vi "NI VeriStand - Update Custom Device Flag.vi"(8 "error in (no error)":errorcluster, 10 "Is Custom Device Active?":bool, 11 "Device Ref in":T1 format="%.0x") -> (0 "error out":errorcluster, 3 "Device Ref out":T1 format="%.0x")   [LabVIEW 2020, in "Custom Device API.lvlib"]
doc: "Flags a custom device as active or inactive."
uses:
  <vilib>/NI VeriStand/Custom Device API/Custom Device API.lvlib
  <vilib>/NI VeriStand/Custom Device API/Custom Device Item Ref.ctl
  <vilib>/NI VeriStand/Custom Device API/Custom Device Status.ctl
  380d47f6-5555-4561-b896-d523444e7594.vi
  <vilib>/NI VeriStand/Custom Device API/Custom Device Offline Path.vi
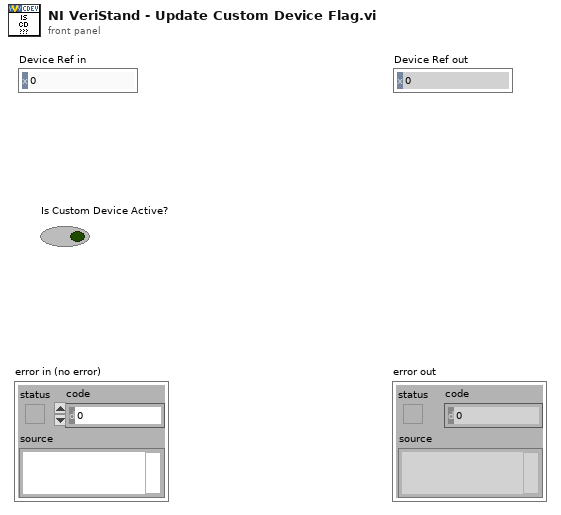
[diagram p1: front panel]
types:
  T1 = typedef "Custom Device API.lvlib/Custom Device Item Ref.ctl" = u64
  T2 = typedef "Custom Device API.lvlib/Custom Device Status.ctl" = enum32{"Not a CD", "Active CD", "Inactive CD"}
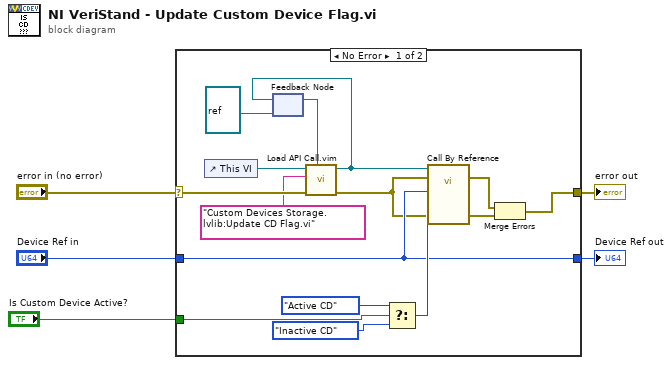
[diagram p0: block diagram]
diagram:
  n1 = case shown="No Error" "error in (no error)" {
    selector: "error in (no error)" -> [w11 w21]
    tunnel: [w19 w21] -> w5
    tunnel: "Device Ref in" -> [w14 w22]
    tunnel: "Is Custom Device Active?" -> [w16 _]
    tunnel: [w14 w22] -> w1
    frame No Error {
      n2 = control-ref of="This VI"() -> (w12:refnum<vi>)
      n3 = feedback #1(refnum<vi> refnum ("type specifier VI Refnum (for type only)")) -> (w13:refnum<vi>)
      n4 = call "Load API Call.vim"("VI reference in"=w13, "error in (no error)"=w11, "VI qualified name"="Custom Devices Storage.lvlib:Update CD Flag.vi", "Caller VI ref"=w12) -> ("error out"=w10:errorcluster, "VI reference"=w9:refnum<vi>)  [unwired: 6 in]
      n5 = feedback-in #1(w9) -> ()
      n6 = Select(t=Custom_Device_Status."Active CD" ("CD Status"), s=w16, f=Custom_Device_Status."Inactive CD" ("CD Status")) -> (s? t:f=w17:T2)
      n7 = call-by-ref "?"(reference=w9, error in=w10, 8:"error in (no error)"=w10, "CD Status"=w17, "Item Reference"=w14) -> (error out=w6:errorcluster, 0:"error out"=w20:errorcluster)  [unwired: 7 in, 2 out]
      n8 = Merge Errors(w6, w20) -> (w19:errorcluster)
    }
    frame Error {
    }
  }
  "Device Ref out" <- w1
  "error out" <- w5
